vi "List post metadata parameters as string.vi"(0 "section names":string[](array[string])=["system control", "file information", "sample information", "cantilever information", "XYZ piezos", "mapping parameters"], 5 "error in (no error)":errorcluster, 8 "appended array":T1[](array[typedef])) -> (14 "Pre Metadat Fcurve":string, 19 "error out":errorcluster)   [LabVIEW 2019, in "metadata.lvclass"]
uses:
  metadata.lvclass
  Metadata output --cluster.ctl
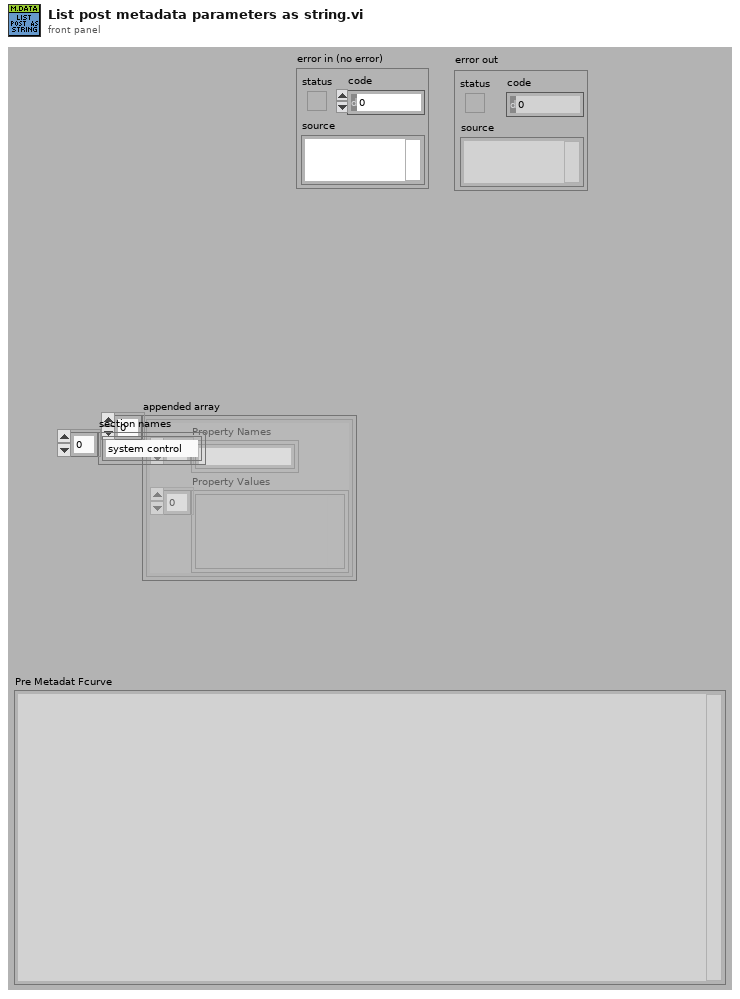
[diagram p1: front panel]
types:
  T1 = typedef "metadata.lvclass/Metadata output --cluster.ctl" = cluster{"Property Names":string[], "Property Values":variant[]}
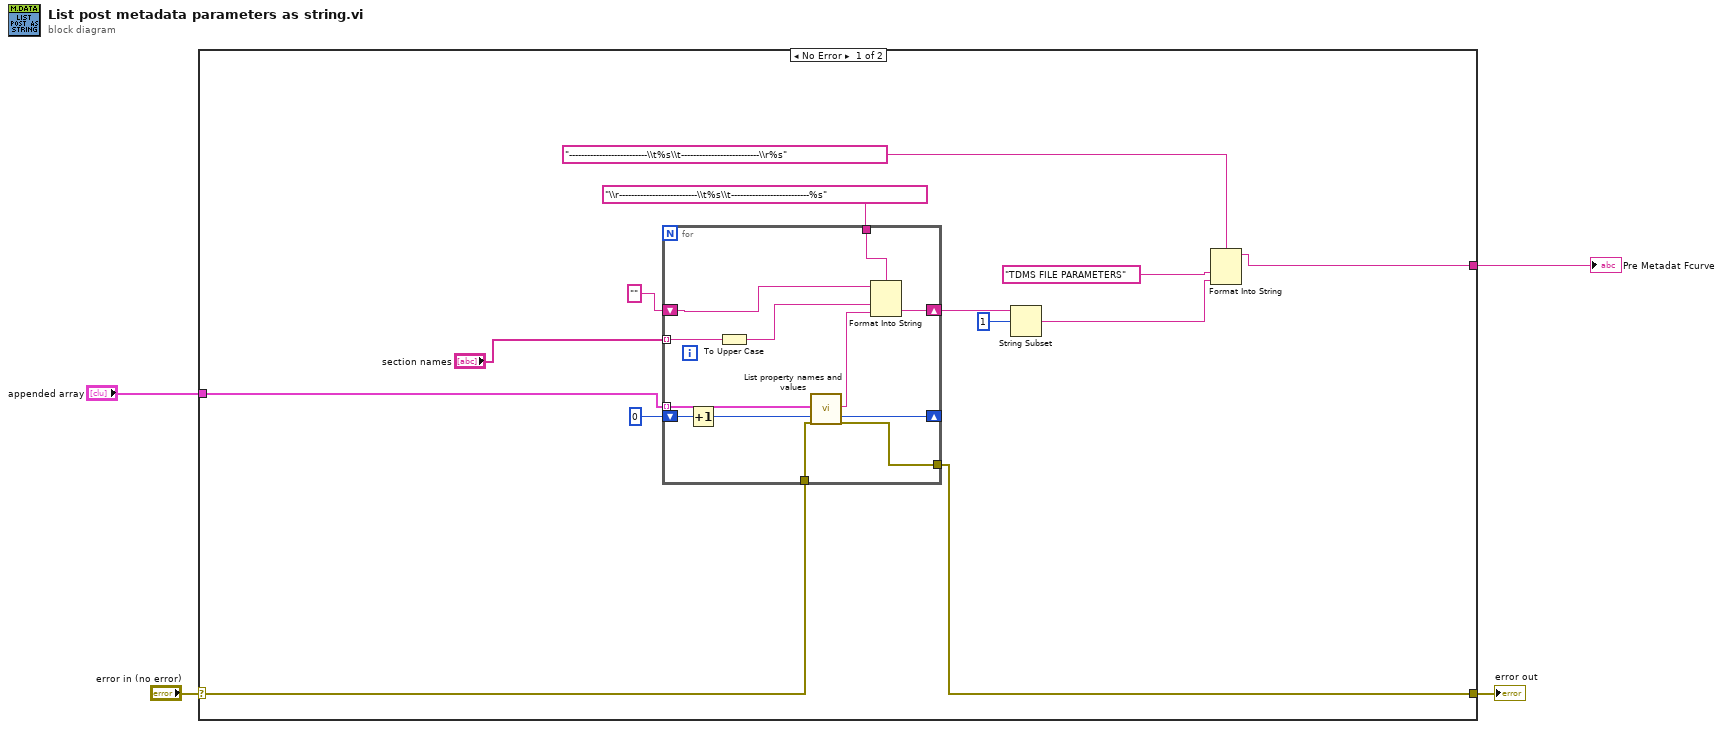
[diagram p0: block diagram]
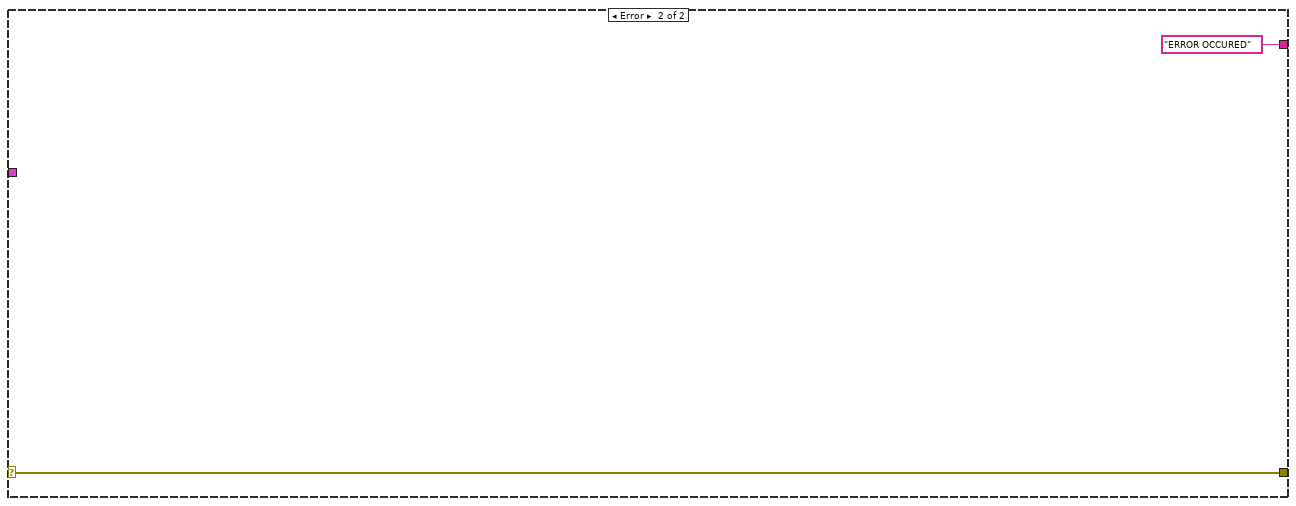
[diagram p2: hidden frame]
diagram:
  n1 = case shown="No Error" "error in (no error)" {
    selector: "error in (no error)" -> [w7 w31]
    tunnel: [w6 w31] -> w3
    tunnel: "appended array" -> [w9 _]
    tunnel: [w8 "ERROR OCCURED"] -> w1
    frame No Error {
      n2 = for {
        tunnel: w9 -> [w29] mode=indexing
        shift-right: [w24] -> w16
        shift-left: "" -> [w20]
        shift-right: [w28] -> _
        shift-left: 0 ("Last index") -> [w27]
        tunnel: [w26] -> w6
        tunnel: w7 -> [w25]
        tunnel: "\\r--------------------------\\t%s\\t--------------------------%s" ("List of property names") -> [w23]
        tunnel: "section names" -> [w18] mode=indexing
        n3 = Increment(x=w27) -> (x+1=w22:i32)
        n4 = To Upper Case(1:w18) -> (0:w19:string)
        n5 = call "List property names and values.vi"("Metadata"=w29, "Prev eindex"=w22, "error in (no error)"=w25) -> ("List of property names"=w21:string, "Last index"=w28:i32, "error out"=w26:errorcluster)  [unwired: 14 in]
        n6 = Format Into String(format string=w23, initial string=w20, w19, w21) -> (resulting string=w24:string)  [unwired: 1 in, 1 out]
      }
      n7 = String Subset(string=w16, offset (0)=1) -> (substring=w11:string)  [unwired: 1 in]
      n8 = Format Into String(format string="--------------------------\\t%s\\t--------------------------\\r%s" ("List of property names"), "TDMS FILE PARAMETERS" ("input 1"), w11) -> (resulting string=w8:string)  [unwired: 2 in, 1 out]
    }
    frame Error {
    }
  }
  "error out" <- w3
  "Pre Metadat Fcurve" <- w1
